vi "Update Graphs.vi"(8 "error in (no error)":errorcluster, 11 "MFC in":refnum<class "Valve.lvclass">) -> (0 "error out":errorcluster, 3 "MFC out":refnum<class "Valve.lvclass">)   [LabVIEW 2013, in "Valve.lvlib" / "Valve.lvclass"]
uses:
  Valve.lvclass
  Valve.lvclass/Valve.ctl
  Read Graph History.vi
  Read Graph.vi
  PluginInterface/PluginInterface.lvlibp/PluginInterfaceClass/Read TDMS.vi
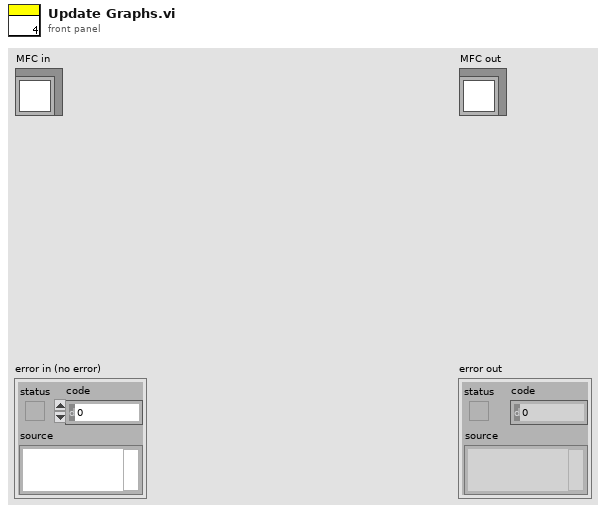
[diagram p1: front panel]
types:
  T1 = cluster{"output array":dbl[], "output array":dbl[]}
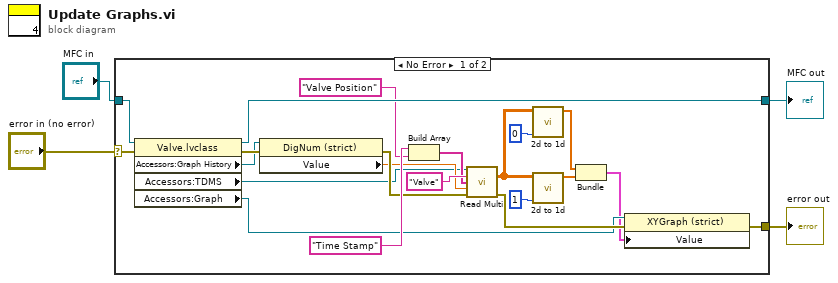
[diagram p0: block diagram]
diagram:
  n1 = case shown="No Error" "error in (no error)" {
    selector: "error in (no error)" -> [w21 w27]
    tunnel: [w6 w27] -> w1
    tunnel: [w24 w26] -> w2
    tunnel: "MFC in" -> [w25 w26]
    frame No Error {
      n2 = property class="Valve.lvclass"(reference=w25, error in=w21) -> (reference out=w24:refnum<class "Valve.lvclass">, error out=w20:errorcluster, "Accessors:Graph History"=w14:refnum<vi>, "Accessors:TDMS"=w15:refnum<k34>, "Accessors:Graph"=w12:refnum<vi>)
      n3 = property class="DigNum (strict)"(reference=w14, error in=w20) -> (error out=w19:errorcluster, "Value"=w16:dbl)  [unwired: 1 out]
      n4 = Build Array("Time Stamp" ("Channel"), "Valve Position" ("string")) -> (w17:string[])
      n5 = call "Read Multi.vi"("tdms file in"=w15, "group"="Valve", "Channel"=w17, "Numeric"=w16, "error in (no error)"=w19) -> ("Array"=w7:dbl[][], "error out"=w13:errorcluster)  [unwired: 7 in, 2 out]
      n6 = call "2d to 1d.vi"("index"=0, "array"=w7) -> ("output array"=w8:dbl[])  [unwired: 9 in]
      n7 = call "2d to 1d.vi"("index"=1, "array"=w7) -> ("output array"=w9:dbl[])  [unwired: 9 in]
      n8 = Bundle("output array"=w8, "output array"=w9) -> (w5:T1)  [unwired: 1 in]
      n9 = property class="XYGraph (strict)"(reference=w12, error in=w13, "Value"=w5) -> (error out=w6:errorcluster)  [unwired: 1 out]
    }
    frame Error {
    }
  }
  "error out" <- w1
  "MFC out" <- w2
